vi "Get IMAQ Ref Index.vi"(0 "Image Idx":i32, 11 "Error In":errorcluster) -> (4 "Image Ref":T1, 15 "Error Out":errorcluster)   [LabVIEW 2020]
uses:
  <vilib>/vision/Image Controls.llb/IMAQ Image.ctl
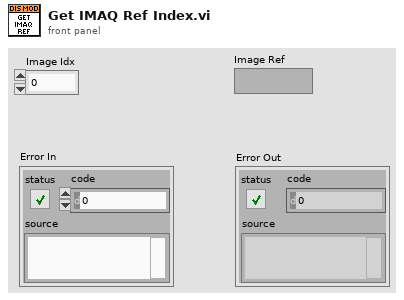
[diagram p1: front panel]
types:
  T1 = typedef "IMAQ Image.ctl" = refnum<image>
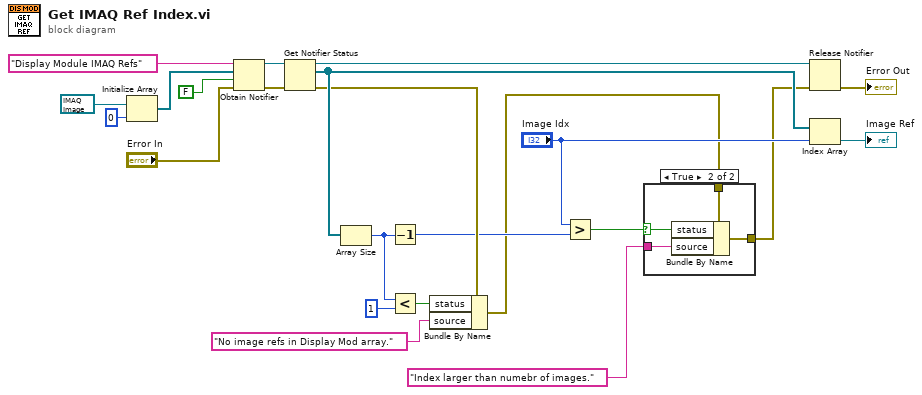
[diagram p0: block diagram]
diagram:
  n1 = Initialize Array(T1 refnum ("New Image"), 0 ("dimension size")) -> (w19:T1[])
  n2 = Obtain Notifier(name (unnamed)="Display Module IMAQ Refs", notification data type=w19, create if not found? (T)=FALSE, error in (no error)="Error In") -> (notifier out=w18:refnum<notifier>, error out=w17:errorcluster)  [unwired: 1 out]
  n3 = Get Notifier Status(notifier=w18, error in (no error)=w17) -> (notifier out=w16:refnum<notifier>, current notification=w14:T1[], error out=w13:errorcluster)  [unwired: 2 out]
  n4 = Array Size(array=w14) -> (size(s)=w9:i32)
  n5 = Decrement(x=w9) -> (x-1=w8:i32)
  n6 = Less?(x=w9, y=1) -> (x < y?=w11:bool)
  n7 = Bundle By Name(cluster=w13, "status"=w11, "source"="No image refs in Display Mod array.") -> (w6:errorcluster)
  n8 = Greater?(x="Image Idx", y=w8) -> (0:w4:bool)
  n9 = case shown="True" w4 {
    selector: w4 -> [_ w26]
    tunnel: w6 -> [w24 w28]
    tunnel: "Index larger than numebr of images." ("source") -> [_ w27]
    tunnel: [w24 w25] -> w3
    frame False {
    }
    frame True {
      n10 = Bundle By Name(cluster=w28, "status"=w26, "source"=w27) -> (w25:errorcluster)
    }
  }
  n11 = Release Notifier(notifier=w16, error in (no error)=w3) -> (error out=→"Error Out":errorcluster)  [unwired: 1 in, 2 out]
  n12 = Index Array(array=w14, index="Image Idx") -> (element=→"Image Ref":T1)
